vi "SDI-12 Continuous Operations 2015.vi"(0 "RS232 Port In":refnum<visa-resource-name>="COM11", 1 "file directory (dialog if empty)":path=path "D:/Cascade/Raw Data files", 5 "Sensor Address In":string="0", 11 "Error In (No Error)":errorcluster, 12 "Save File":bool) -> (3 "new file path (Not A Path if cancelled)":path, 6 "Address Out":string="a" caption="sensor address out", 8 "Temperature":cluster{"Y":dbl[], "Y":dbl[]}[](graph), 10 "Sonde Data Display":T1, 13 "Measurements Out":dbl[](array[numeric]), 14 "Array":timestamp[](array[timestamp]), 15 "Error Out":errorcluster)   [LabVIEW 2015]
doc: "A general set of examples of the SDI-12 API for a generic sensor. A tab control separates each example, and contains the following examples:\n1. Read Single.\n2. Read Multiple.\n3. Acknowledge Active.\n4. Change Address.\n5. Address Query.\n6. Send Identification."
uses:
  SDI-12/Sonde Vertical Graph.ctl
  Waterloo DAQ/controls/Vertical Chart.ctl
  <vilib>/Utility/file.llb/Write Delimited Spreadsheet (string).vi
  <vilib>/Utility/file.llb/Write Delimited Spreadsheet (DBL).vi
  SDI-12/SDI-12.lvlib
panel:
  out "Number of Measurements Out":i32
  in  "Measurement Type In (Normal)":i32(ring)=1 items=["Normal", "Concurrent", "Continuous"]
  out "Parameter Out":i32(ring) items=["0", "1", "2", "3", "4", "5", "6", "7", "8", "9"]
  in  "Parameter In (0)":i32(ring) items=["0", "1", "2", "3", "4", "5", "6", "7", "8", "9"]
  in  "CRC (False)":bool
  out "CRC Out":bool
  out "Measurement Type Out":i32(ring) items=["Normal", "Concurrent", "Continuous"]
  out "Time (s)":dbl
  in  "stop":bool
  out "counter":i32
  out "start time":timestamp
  # "deg C"
  # "pH"
  # "specific conductance"
  # "salinity"
  # "DO % saturation"
  # "DO mg/L"
  # "ORP"
  # "depth"
  # "battery"
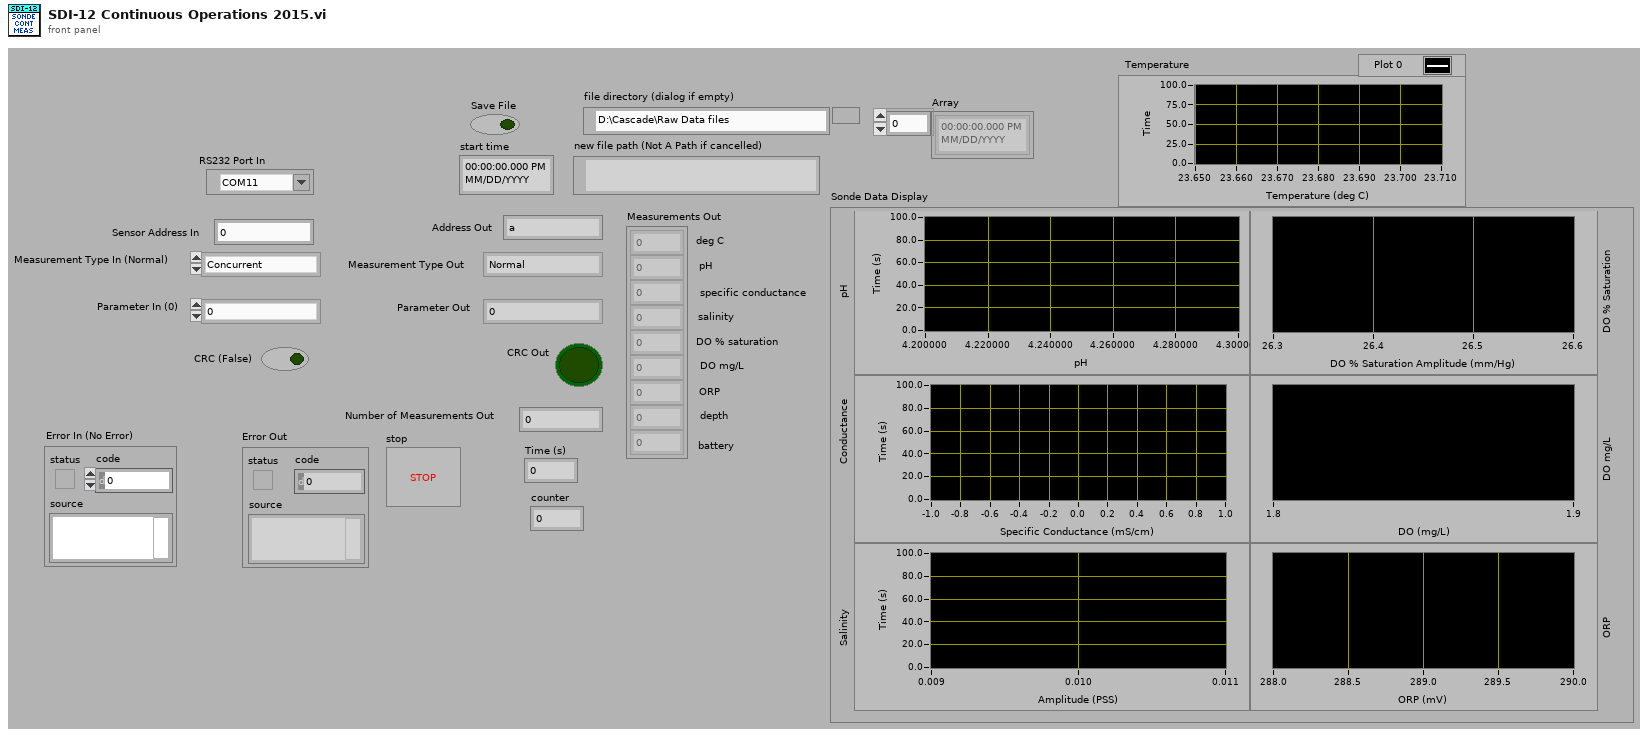
[diagram p1: front panel]
types:
  T1 = typedef "Sonde Vertical Graph.ctl" = cluster{"pH":T2, "Conductance":T2, "Salinity":T2, "DO % Saturation":T2, "DO mg/L":T2, "ORP":T2}
  T2 = typedef "Vertical Chart.ctl" = cluster{"Y":dbl[], "Y":dbl[]}[]
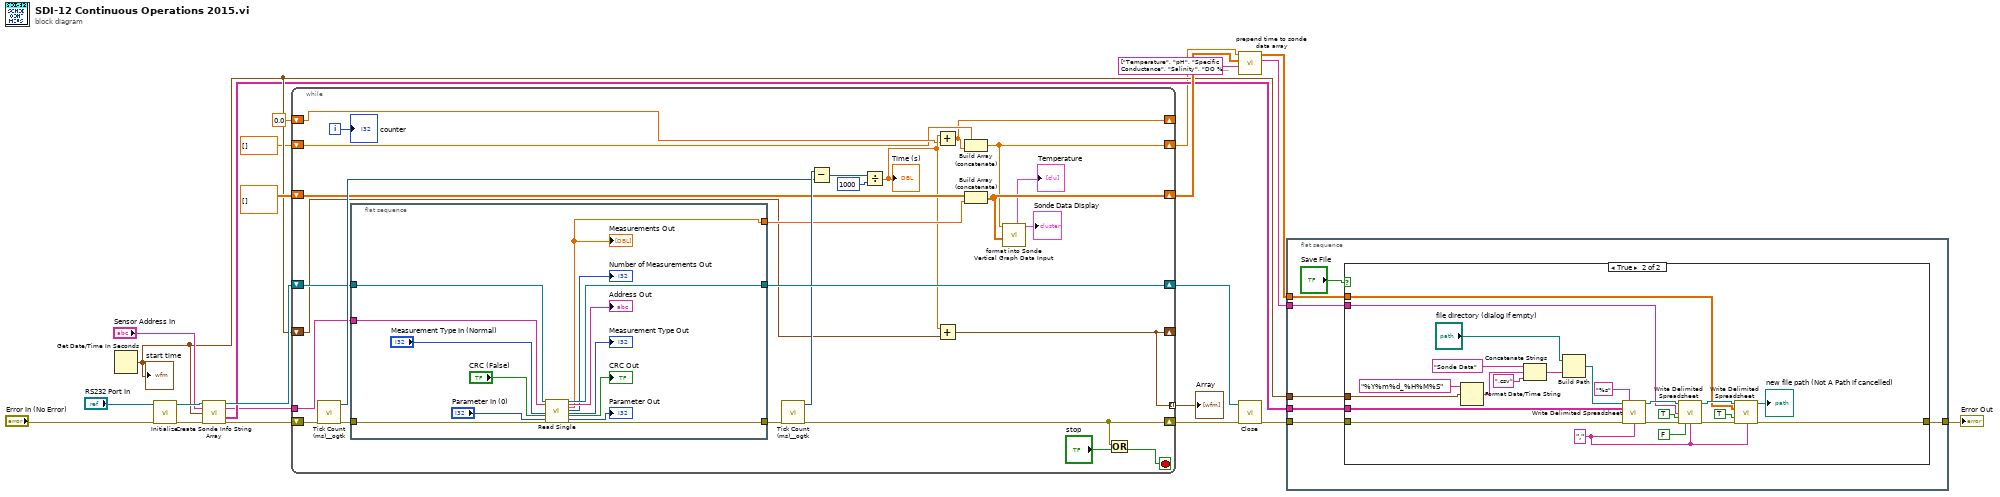
[diagram p0: block diagram]
diagram:
  n1 = Get Date/Time In Seconds() -> (seconds since 1Jan1904=w8:timestamp)
  "start time" <- w8
  n2 = call "Initialize.vi"("Error In (No Error)"="Error In (No Error)", "RS232 Port In"="RS232 Port In") -> ("Error Out"=w19:errorcluster, "RS232 Port Out"=w18:refnum<visa-resource-name>)  [unwired: 8 in]
  n3 = call "Create Sonde Info String Array.vi"("VISA Refnum in"=w18, "Sensor Address In"="Sensor Address In", "seconds since 1Jan1904"=w8, "error in (no error)"=w19) -> ("VISA Refnum out"=w17:refnum<visa-resource-name>, "Address Out"=w6:string, "Array"=w7:string[][], "error out"=w16:errorcluster)  [unwired: 8 in]
  n4 = while {
    shift-right: [w49] -> w20
    shift-left: w17 -> [w42]
    shift-right: [w24] -> w21
    shift-left: w16 -> [w41]
    shift-right: [w36] -> w13
    shift-left: dbl[][] [] -> [w37]
    tunnel: [w34] -> w14 mode=indexing
    shift-right: [w34] -> _
    shift-left: w8 -> [w35]
    shift-right: [w32] -> w3
    shift-left: dbl[] [] -> [w28]
    tunnel: w6 -> [w33]
    shift-right: [w27] -> _
    shift-left: 0.0 -> [w29]
    i -> [w39]
    stop <- w25 stop-if-true
    n5 = call <userlib>:"Tick Count (ms)__ogtk.vi"("error in (no error)"=w41) -> ("error out"=w47:errorcluster, "millisecond timer value"=w45:u32)  [unwired: 9 in]
    n6 = flat-sequence {
      tunnel: [w63] -> w49
      tunnel: [w62] -> w48
      tunnel: w47 -> [w53]
      tunnel: w42 -> [w52]
      tunnel: [w51] -> w38
      tunnel: w33 -> [w50]
      frame #0 {
        n7 = call "Read Single.vi"("RS232 Port In"=w52, "Sensor Address In"=w50, "Measurement Type In (Normal)"="Measurement Type In (Normal)", "CRC (False)"="CRC (False)", "Parameter In (0)"="Parameter In (0)", "Error In (No Error)"=w53) -> ("RS232 Port Out"=w63:refnum<visa-resource-name>, "Sensor Address Out"=→"Address Out":string, "Measurements Out"=w51:dbl[], "Number of Measurements Out"=→"Number of Measurements Out":i32, "Measurement Type Out"=→"Measurement Type Out":i32, "CRC Out"=→"CRC Out":bool, "Parameter Out"=→"Parameter Out":i32, "Error Out"=w62:errorcluster)  [unwired: 14 in]
        "Measurements Out" <- w51
      }
    }
    n8 = call <userlib>:"Tick Count (ms)__ogtk.vi"("error in (no error)"=w48) -> ("error out"=w24:errorcluster, "millisecond timer value"=w46:u32)  [unwired: 9 in]
    n9 = Subtract(x=w46, y=w45) -> (x-y=w44:u32)
    n10 = Divide(x=w44, y=u32 1000) -> (x/y=w30:dbl)
    "Time (s)" <- w30
    n11 = Add(x=w30, y=w29) -> (x+y=w27:dbl)
    n12 = Add(x=w30, y=w35) -> (x+y=w34:timestamp)
    n13 = Build Array (concatenate)(w28, w27) -> (w32:dbl[])
    n14 = Build Array (concatenate)(w37, w38) -> (w36:dbl[][])
    n15 = call "format into Sonde Vertical Graph Data Input.vi"("Sonde Measurement Array"=w36, "Time Array"=w32) -> ("Sonde Data Display out"=→"Sonde Data Display":T1, "Temperature"=→"Temperature":cluster{"X":dbl[], "Y":dbl[]}[])  [unwired: 8 in]
    n16 = Or(x=w24, y="stop") -> (x .or. y?=w25:bool)
    "counter" <- w39
  }
  "Array" <- w14
  n17 = call "prepend time to sonde data array.vi"("Measurement Labels"=string[] ["Temperature", "pH", "Specific Conductance", "Salinity", "DO % saturation", "DO", "ORP", "depth", "battery"], "Sonde\nData Array"=w13, "Time Array"=w3) -> ("Header Array"=w5:string[], "Data Array"=w10:dbl[][])  [unwired: 7 in]
  n18 = call "Close.vi"("Error In (No Error)"=w21, "RS232 Port In"=w20) -> ("Error Out"=w12:errorcluster)  [unwired: 9 in]
  n19 = flat-sequence {
    tunnel: w12 -> [w70]
    tunnel: [w69] -> w11
    tunnel: w5 -> [w67]
    tunnel: w10 -> [w66]
    tunnel: w8 -> [w65]
    tunnel: w7 -> [w64]
    frame #0 {
      n20 = case shown="True" "Save File" {
        tunnel: [w71 w91] -> w69
        tunnel: w70 -> [w71 w76]
        tunnel: w67 -> [_ w72]
        tunnel: w66 -> [_ w89]
        tunnel: w65 -> [_ w83]
        tunnel: w64 -> [_ w74]
        frame False {
        }
        frame True {
          w73 = "," ("delimiter (\\t)")
          n21 = Format Date/Time String(time format string (%c)="%Y%m%d_%H%M%S", seconds (now)=w83) -> (date/time string=w82:string)  [unwired: 1 in]
          n22 = Concatenate Strings("Sonde Data" ("name or relative path"), w82, ".csv" ("string")) -> (w84:string)
          n23 = Build Path(base path="file directory (dialog if empty)", name or relative path=w84) -> (appended path=w79:path)
          n24 = call-poly <vilib>:"Write Delimited Spreadsheet.vi"("file path (dialog if empty)"=w79, "format (%s)"="%s" ("format (%.3f)"), "2D data"=w74, "error in (no error)"=w76, "delimiter (\\t)"=w73) -> ("new file path (Not A Path if cancelled)"=w78:path, "error out"=w75:errorcluster)  [unwired: 9 in]
          n25 = call-poly <vilib>:"Write Delimited Spreadsheet.vi"("file path (dialog if empty)"=w78, "1D data"=w72, "append to file? (F)"=TRUE, "error in (no error)"=w75, "transpose? (F)"=FALSE, "delimiter (\\t)"=w73) -> ("new file path (Not A Path if cancelled)"=w93:path, "error out"=w92:errorcluster)  [unwired: 8 in]
          n26 = call-poly <vilib>:"Write Delimited Spreadsheet.vi"("file path (dialog if empty)"=w93, "2D data"=w89, "append to file? (F)"=TRUE, "error in (no error)"=w92, "delimiter (\\t)"=w73) -> ("new file path (Not A Path if cancelled)"=→"new file path (Not A Path if cancelled)":path, "error out"=w91:errorcluster)  [unwired: 9 in]
        }
      }
    }
  }
  "Error Out" <- w11
